vi "Update Time Trace.vi"(1 "Channel Index":i32, 2 "Time (s)":dbl[](array[numeric])) -> ()   [LabVIEW 2022 SP3]
uses:
  Globals/Meas_global.vi
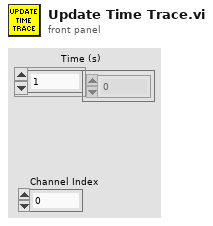
[diagram p1: front panel]
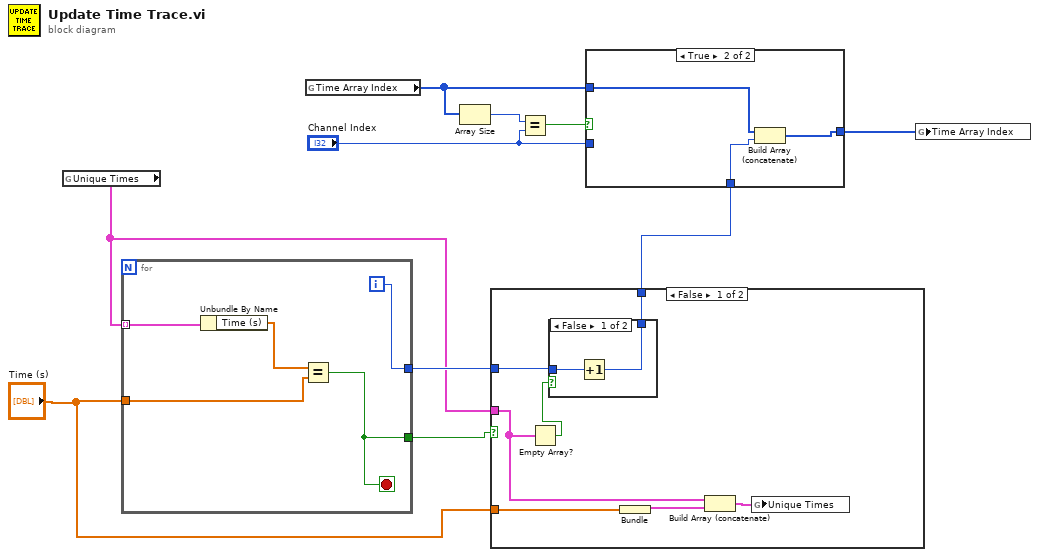
[diagram p0: block diagram]
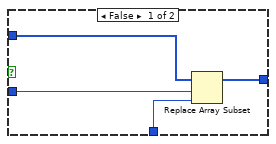
[diagram p2: hidden frame]
diagram:
  n1 = global read "Meas_global.vi" "Unique Times"() -> (w6:cluster{"Time (s)":dbl[]}[])
  n2 = for {
    tunnel: w6 -> [w15] mode=indexing
    tunnel: "Time (s)" -> [w13]
    tunnel: [w12] -> w8
    tunnel: [w11] -> w7
    i -> [w11]
    stop <- w12 stop-if-true
    n3 = Unbundle By Name(w15) -> ("Time (s)"=w14:dbl[])
    n4 = Equal?(x=w14, y=w13) -> (x = y?=w12:bool)
  }
  n5 = global read "Meas_global.vi" "Time Array Index"() -> (w4:i32[])
  n6 = Array Size(array=w4) -> (size(s)=w2:i32)
  n7 = case shown="False" w8 {
    tunnel: w7 -> [w22 w26]
    tunnel: [w21 w26] -> w9
    tunnel: "Time (s)" -> [w18 _]
    tunnel: w6 -> [w17 _]
    frame False {
      n8 = Empty Array?(array=w17) -> (empty?=w16:bool)
      n9 = case shown="False" w16 {
        tunnel: w22 -> [w24 w25]
        tunnel: [w23 w25] -> w21
        frame False {
          n10 = Increment(x=w24) -> (x+1=w23:i32)
        }
        frame True {
        }
      }
      n11 = Bundle("Time (s)"=w18) -> (w20:cluster{"Time (s)":dbl[]})  [unwired: 1 in]
      n12 = Build Array (concatenate)(w17, w20) -> (w19:cluster{"Time (s)":dbl[]}[])
      n13 = global write "Meas_global.vi" "Unique Times"(w19) -> ()
    }
    frame True {
    }
  }
  n14 = Equal?(x=w2, y="Channel Index") -> (x = y?=w1:bool)
  n15 = case shown="True" w1 {
    tunnel: [w30 w31] -> w10
    tunnel: w9 -> [w29 w33]
    tunnel: w4 -> [w28 w32]
    tunnel: "Channel Index" -> [w27 _]
    frame False {
      n16 = Replace Array Subset(array=w28, new element=w29, index=w27) -> (w30:i32[])
    }
    frame True {
      n17 = Build Array (concatenate)(w32, w33) -> (w31:i32[])
    }
  }
  n18 = global write "Meas_global.vi" "Time Array Index"(w10) -> ()
